vi "eFGV - Palette.vi"(6 "eFGV States":T1, 8 "Error In":errorcluster, 11 "Enum":T2(ring)) -> (0 "Error Out":errorcluster, 3 "Enum REF":refnum<user-event>)   [LabVIEW 2020]
uses:
  Control/State - eFGV.ctl
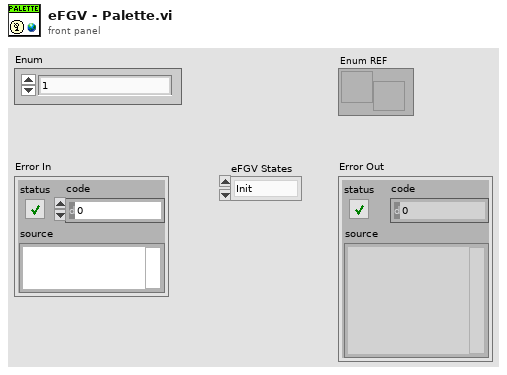
[diagram p1: front panel]
types:
  T1 = typedef "State - eFGV.ctl" = enum16{"Init", "Read", "Write", "Exit"}
  T2 = enum32{"1", "2", "3", "4", "5", "6", "7", "8", "9"}
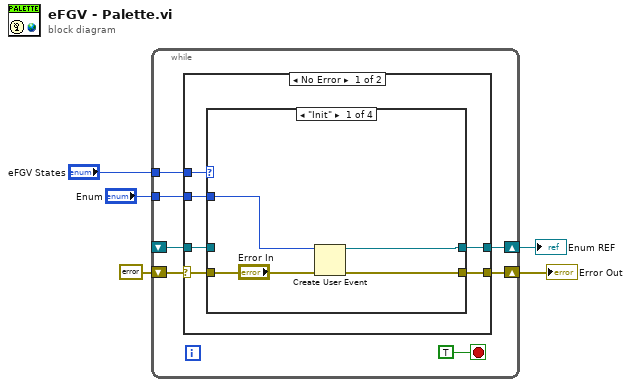
[diagram p0: block diagram]
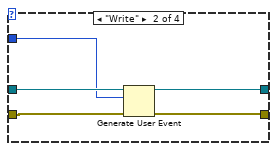
[diagram p2: hidden frame]
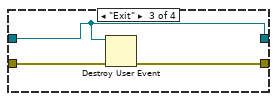
[diagram p3: hidden frame]
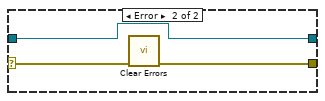
[diagram p5: hidden frame]
diagram:
  n1 = while {
    tunnel: "eFGV States" -> [w9]
    shift-right: [w11] -> w5
    shift-left: errorcluster {"status"=FALSE, "code"=0, "source"=""} ("error out") -> [w12]
    shift-right: [w8] -> w3
    shift-left: _ -> [w7]
    tunnel: "Enum" -> [w6]
    stop <- TRUE stop-if-true
    n2 = case shown="No Error" w12 {
      selector: w12 -> [w18 w34]
      tunnel: [w17 w35] -> w11
      tunnel: w9 -> [w16 _]
      tunnel: [w15 w33] -> w8
      tunnel: w7 -> [w14 w33]
      tunnel: w6 -> [w13 _]
      frame No Error {
        n3 = case shown="\"Init\"" w16 {
          tunnel: w18 -> [w22 w26 w30 w32]
          tunnel: [w21 w27 w29 w32] -> w17
          tunnel: [w20 w25 w28 w31] -> w15
          tunnel: w14 -> [_ w24 w28 w31]
          tunnel: w13 -> [w19 w23 _ _]
          frame "Init" {
            n4 = Create User Event(user event datatype=w19, error in=w22) -> (user event=w20:refnum<user-event>, error out=w21:errorcluster)
          }
          frame "Write" {
            n5 = Generate User Event(user event=w24, event data cluster=w23, error in=w26) -> (user event out=w25:refnum<user-event>, error out=w27:errorcluster)  [unwired: 1 in]
          }
          frame "Exit" {
            n6 = Destroy User Event(user event=w28, error in=w30) -> (error out=w29:errorcluster)
          }
          frame "Read" {
          }
        }
      }
      frame Error {
        n7 = call <vilib>:"Clear Errors.vi"("error in (no error)"=w34) -> ("error out"=w35:errorcluster)  [unwired: 5 in, 1 out]
      }
    }
  }
  "Error Out" <- w5
  "Enum REF" <- w3
